vi "DecodeData.vi"(11 "Input Data":string) -> (1 "Angular Step Width":dbl format="%.2f", 2 "Starting Angle":dbl format="%.2f", 3 "Decoded Data":dbl[](array[numeric]) format="%.2f")   [LabVIEW 2009]
panel:
  out "NumberData":u16
  out "Scaling Offset":dbl format="%.2f"
  out "Scaling Factor":dbl format="%.2f"
  out "subarray":string[](array[string])
  out "Array":string[](array[string])
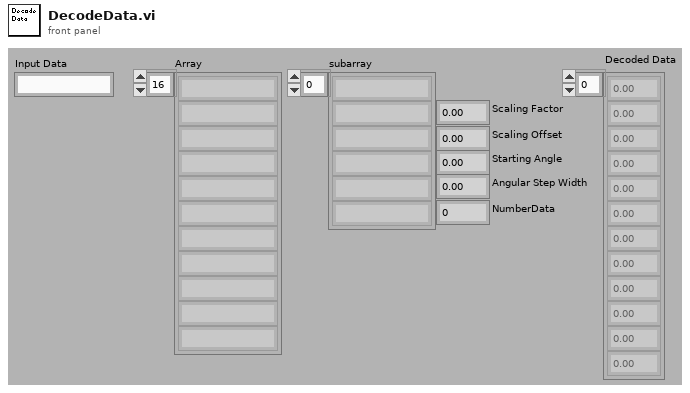
[diagram p1: front panel]
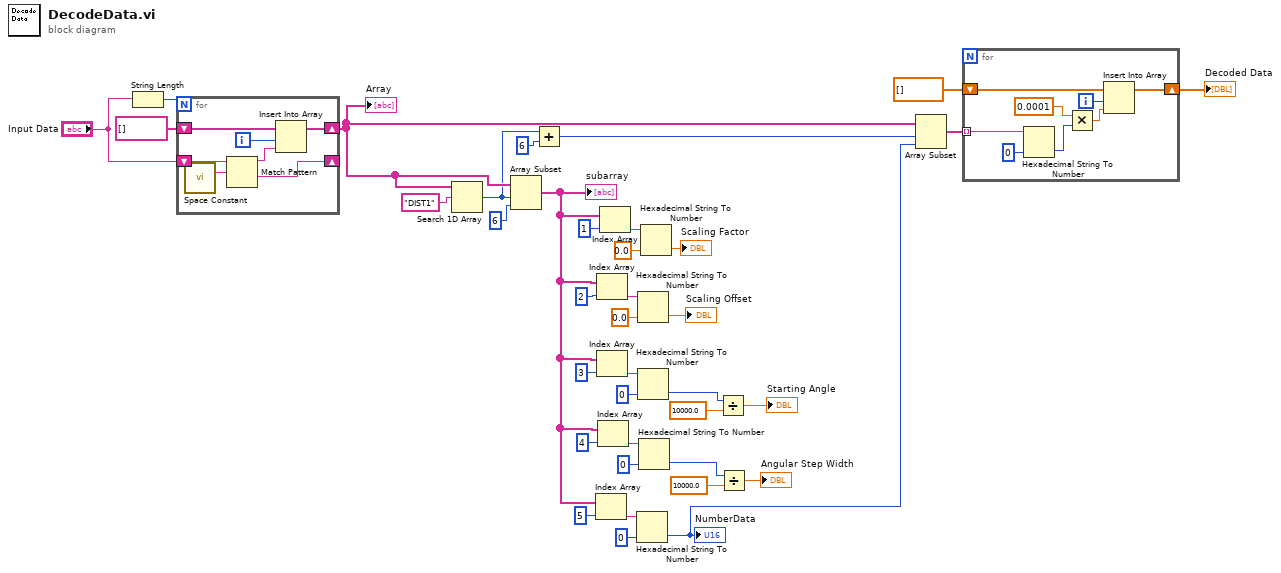
[diagram p0: block diagram]
diagram:
  n1 = String Length(string="Input Data") -> (length=w37:i32)
  n2 = for {
    N: w37 -> [_]
    shift-right: [w42] -> _
    shift-left: "Input Data" -> [w44]
    shift-right: [w40] -> w10
    shift-left: string[] [] -> [w41]
    i -> [w38]
    n3 = call <vilib>:"Space Constant.vi"() -> ("String"=w43:string)
    n4 = Match Pattern(string=w44, regular expression=w43) -> (before substring=w39:string, after substring=w42:string)  [unwired: 1 in, 2 out]
    n5 = Insert Into Array(array=w41, index=w38, new element=w39) -> (w40:string[])
  }
  "Array" <- w10
  n6 = Search 1D Array(1D array=w10, element="DIST1") -> (index of element=w6:i32)  [unwired: 1 in]
  n7 = Array Subset(array=w10, index=w6, length=6) -> (w9:string[])
  "subarray" <- w9
  n8 = Add(x=w6, y=6) -> (x+y=w14:i32)
  n9 = Index Array(array=w9, index=5) -> (element=w20:string)
  n10 = Index Array(array=w9, index=2) -> (element=w29:string)
  n11 = Index Array(array=w9, index=3) -> (element=w26:string)
  n12 = Index Array(array=w9, index=4) -> (element=w23:string)
  n13 = Index Array(array=w9, index=1) -> (element=w33:string)
  n14 = Hexadecimal String To Number(string=w20, default (0uL)=u16 0 ("default (0 U32)")) -> (number=w15:u16)  [unwired: 1 in, 1 out]
  "NumberData" <- w15
  n15 = Hexadecimal String To Number(string=w29, default (0uL)=0.0 ("default (0 U32)")) -> (number=→"Scaling Offset":dbl)  [unwired: 1 in, 1 out]
  n16 = Hexadecimal String To Number(string=w26, default (0uL)=0 ("default (0 U32)")) -> (number=w18:i32)  [unwired: 1 in, 1 out]
  n17 = Hexadecimal String To Number(string=w23, default (0uL)=u16 0 ("default (0 U32)")) -> (number=w3:u16)  [unwired: 1 in, 1 out]
  n18 = Hexadecimal String To Number(string=w33, default (0uL)=0.0 ("default (0 U32)")) -> (number=→"Scaling Factor":dbl)  [unwired: 1 in, 1 out]
  n19 = Divide(x=w18, y=10000.0) -> (x/y=→"Starting Angle":dbl)
  n20 = Divide(x=w3, y=10000.0) -> (x/y=→"Angular Step Width":dbl)
  n21 = Array Subset(array=w10, index=w14, length=w15) -> (w13:string[])
  n22 = for {
    tunnel: w13 -> [w49] mode=indexing
    shift-right: [w50] -> w11
    shift-left: dbl[] [] -> [w51]
    i -> [w48]
    n23 = Hexadecimal String To Number(string=w49, default (0uL)=u16 0 ("default (0 U32)")) -> (number=w47:u16)  [unwired: 1 in, 1 out]
    n24 = Multiply(x=0.0001, y=w47) -> (x*y=w46:dbl)
    n25 = Insert Into Array(array=w51, index=w48, new element=w46) -> (w50:dbl[])
  }
  "Decoded Data" <- w11
